vi "volts_to_bits_thrs.vi"(11 "Voltage":dbl) -> (3 "Bits":string)   [LabVIEW 2015]
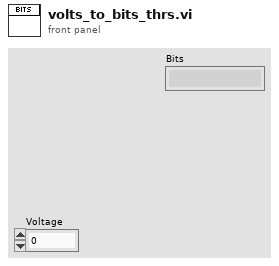
[diagram p1: front panel]
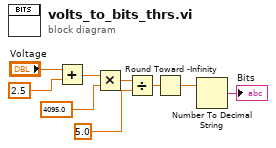
[diagram p0: block diagram]
diagram:
  n1 = Add(x="Voltage", y=2.5) -> (x+y=w7:dbl)
  n2 = Multiply(x=w7, y=4095.0) -> (x*y=w5:dbl)
  n3 = Divide(x=w5, y=5.0) -> (x/y=w3:dbl)
  n4 = Round Toward -Infinity(1:w3) -> (0:w2:dbl)
  n5 = Number To Decimal String(number=w2) -> (decimal integer string=→"Bits":string)  [unwired: 1 in]
